vi "test_read-nmea-data2.vi"() -> ()   [LabVIEW 2019] (continued)
F9P\t\t\n15:11:09.78\tF9P\t\t\n15:11:09.80\tF9P\t\t\n15:11:09.82\tF9P\t\t\n15:11:09.84\tF9P\t\t\n15:11:09.86\tF9P\t\t\n15:11:09.88\tF9P\t\t\n15:11:09.90\tF9P\t\t\n15:11:09.92\tF9P\t\t\n15:11:09.94\tF9P\t\t\n15:11:09.96\tF9P\t\t\n15:11:09.98\tF9P\t\t\n15:11:10.00\tF9P\t\t\n15:11:10.02\tF9P\t\t\n15:11:10.04\tF9P\t\t\n15:11:10.06\tF9P\t\t\n15:11:10.08\tF9P\t\t\n15:11:10.10\tF9P\t\t\n15:11:10.12\tF9P\t\t\n15:11:10.14\tF9P\t\t\n15:11:10.16\tF9P\t\t\n15:11:10.18\tF9P\t\t\n15:11:10.20\tF9P\t\t\n15:11:10.22\tF9P\t\t\n15:11:10.24\tF9P\t\t\n15:11:10.26\tF9P\t$GNRMC,061112.00,A,3723.54417,N,12656.89832,E,2.532,132.14,250720,,,A,V*06\n\t\n15:11:10.28\tF9P\t$GNVTG,132.14,T,,M,2.532,N,4.690,K,A*2B\n\t\n15:11:10.30\tF9P\t$GNGGA,061112.00,3723.54417,N,12656.89832,E,1,12,0.68,52.3,M,18.5,M,,*7A\n\t\n15:11:10.32\tF9P\t$GNGSA,A,3,12,06,19,05,17,09,02,,,,,,1.27,0.68,1.08,1*07\n\t\n15:11:10.34\tF9P\t$GNGSA,A,3,85,71,84,,,,,,,,,,1.27,0.68,1.08,2*06\n\t\n15:11:10.36\tF9P\t$GNGSA,A,3,36,19,11,04,09,12,,,,,,,1.27,0.68,1.08,3*03\n\t\n15:11:10.38\tF9P\t$GNGSA,A,3,14,11,33,,,,,,,,,,1.27,0.68,1.08,4*02\n\t\n15:11:10.40\tF9P\t$GPGSV,3,1,09,02,54,318,43,04,18,044,20,05,37,247,30,06,64,047,30,1*69\n\t\n15:11:10.42\tF9P\t$GPGSV,3,2,09,09,45,074,27,12,24,277,15,17,33,153,38,19,53,157,29,1*6D\n\t\n15:11:10.44\tF9P\t$GPGSV,3,3,09,25,12,307,19,1*55\n\t\n15:11:10.46\tF9P\t$GPGSV,3,1,09,02,54,318,,04,18,044,,05,37,247,16,06,64,047,16,6*6B\n\t\n15:11:10.48\tF9P\t$GPGSV,3,2,09,09,45,074,18,12,24,277,,17,33,153,19,19,53,157,,6*6A\n\t\n15:11:10.50\tF9P\t$GPGSV,3,3,09,25,12,307,,6*5A\n\t\n15:11:10.52\tF9P\t$GLGSV,2,1,08,69,12,031,,70,72,041,,71,51,205,21,72,03,209,,1*71\n\t\n15:11:10.54\tF9P\t$GLGSV,2,2,08,77,01,326,,84,20,122,12,85,70,065,24,86,36,330,,1*7E\n\t\n15:11:10.56\tF9P\t$GLGSV,2,1,08,69,12,031,,70,72,041,,71,51,205,18,72,03,209,,3*79\n\t\n15:11:10.58\tF9P\t$GLGSV,2,2,08,77,01,326,,84,20,122,16,85,70,065,19,86,36,330,,3*76\n\t\n15:11:10.60\tF9P\t$GAGSV,2,1,08,02,08,297,08,04,66,118,29,09,32,193,20,11,71,358,25,7*7F\n\t\n15:11:10.62\tF9P\t$GAGSV,2,2,08,12,40,102,20,19,26,045,09,25,09,249,,36,25,308,27,7*74\n\t\n15:11:10.64\tF9P\t$GAGSV,2,1,08,02,08,297,,04,66,118,25,09,32,193,,11,71,358,,2*7B\n\t\n15:11:10.66\tF9P\t$GAGSV,2,2,08,12,40,102,21,19,26,045,,25,09,249,,36,25,308,,2*7C\n\t\n15:11:10.68\tF9P\t$GBGSV,1,1,03,11,50,131,27,14,87,138,28,33,60,219,28,1*4A\n\t\n15:11:10.70\tF9P\t$GBGSV,1,1,03,11,50,131,28,14,87,138,25,33,60,219,,3*40\n\t\n15:11:10.72\tF9P\t$GNGLL,3723.54417,N,12656.89832,E,061112.00,A,A*7A\n\t\n15:11:10.74\tF9P\t\t\n15:11:10.76\tF9P\t\t\n15:11:10.78\tF9P\t\t\n15:11:10.80\tF9P\t\t\n15:11:10.82\tF9P\t\t\n15:11:10.84\tF9P\t\t\n15:11:10.86\tF9P\t\t\n15:11:10.88\tF9P\t\t\n15:11:10.90\tF9P\t\t\n15:11:10.92\tF9P\t\t\n15:11:10.94\tF9P\t\t\n15:11:10.96\tF9P\t\t\n15:11:10.98\tF9P\t\t\n15:11:11.00\tF9P\t\t\n15:11:11.02\tF9P\t\t\n15:11:11.04\tF9P\t\t\n15:11:11.06\tF9P\t\t\n15:11:11.08\tF9P\t\t\n15:11:11.10\tF9P\t\t\n15:11:11.12\tF9P\t\t\n15:11:11.14\tF9P\t\t\n15:11:11.16\tF9P\t\t\n15:11:11.18\tF9P\t\t\n15:11:11.20\tF9P\t\t\n15:11:11.22\tF9P\t\t\n15:11:11.24\tF9P\t\t\n15:11:11.26\tF9P\t$GNRMC,061113.00,A,3723.54360,N,12656.89907,E,2.329,127.33,250720,,,A,V*0A\n\t\n15:11:11.28\tF9P\t$GNVTG,127.33,T,,M,2.329,N,4.313,K,A*28\n\t\n15:11:11.30\tF9P\t$GNGGA,061113.00,3723.54360,N,12656.89907,E,1,12,0.68,51.5,M,18.5,M,,*7E\n\t\n15:11:11.32\tF9P\t$GNGSA,A,3,12,06,19,05,17,09,02,,,,,,1.27,0.68,1.08,1*07\n\t\n15:11:11.34\tF9P\t$GNGSA,A,3,85,71,84,,,,,,,,,,1.27,0.68,1.08,2*06\n\t\n15:11:11.36\tF9P\t$GNGSA,A,3,36,19,11,04,09,12,,,,,,,1.27,0.68,1.08,3*03\n\t\n15:11:11.38\tF9P\t$GNGSA,A,3,14,11,33,,,,,,,,,,1.27,0.68,1.08,4*02\n\t\n15:11:11.40\tF9P\t$GPGSV,3,1,09,02,54,318,33,04,18,044,,05,37,247,29,06,64,047,35,1*61\n\t\n15:11:11.42\tF9P\t$GPGSV,3,2,09,09,45,074,26,12,24,277,26,17,33,153,34,19,53,157,29,1*60\n\t\n15:11:11.44\tF9P\t$GPGSV,3,3,09,25,12,307,20,1*5F\n\t\n15:11:11.46\tF9P\t$GPGSV,3,1,09,02,54,318,,04,18,044,,05,37,247,15,06,64,047,13,6*6D\n\t\n15:11:11.48\tF9P\t$GPGSV,3,2,09,09,45,074,18,12,24,277,,17,33,153,19,19,53,157,,6*6A\n\t\n15:11:11.50\tF9P\t$GPGSV,3,3,09,25,12,307,,6*5A\n\t\n15:11:11.52\tF9P\t$GLGSV,2,1,08,69,12,031,,70,72,041,,71,51,205,22,72,03,209,,1*72\n\t\n15:11:11.54\tF9P\t$GLGSV,2,2,08,77,01,326,,84,20,122,12,85,70,065,24,86,36,330,,1*7E\n\t\n15:11:11.56\tF9P\t$GLGSV,2,1,08,69,12,031,,70,72,041,,71,51,205,17,72,03,209,,3*76\n\t\n15:11:11.58\tF9P\t$GLGSV,2,2,08,77,01,326,,84,20,122,19,85,70,065,18,86,36,330,,3*78\n\t\n15:11:11.60\tF9P\t$GAGSV,2,1,08,02,08,297,08,04,66,118,28,09,32,193,22,11,71,358,26,7*7F\n\t\n15:11:11.62\tF9P\t$GAGSV,2,2,08,12,40,102,21,19,26,045,08,25,09,249,,36,25,308,27,7*74\n\t\n15:11:11.64\tF9P\t$GAGSV,2,1,08,02,08,297,,04,66,118,24,09,32,193,,11,71,358,,2*7A\n\t\n15:11:11.66\tF9P\t$GAGSV,2,2,08,12,40,102,21,19,26,045,,25,09,249,,36,25,308,,2*7C\n\t\n15:11:11.68\tF9P\t$GBGSV,1,1,03,11,50,131,27,14,87,138,25,33,60,219,19,1*45\n\t\n15:11:11.70\tF9P\t$GBGSV,1,1,03,11,50,131,27,14,87,138,23,33,60,219,,3*49\n\t\n15:11:11.72\tF9P\t$GNGLL,3723.54360,N,12656.89907,E,061113.00,A,A*7B\n\t\n15:11:11.74\tF9P\t\t\n15:11:11.76\tF9P\t\t\n15:11:11.78\tF9P\t\t\n15:11:11.80\tF9P\t\t\n15:11:11.82\tF9P\t\t\n15:11:11.84\tF9P\t\t\n15:11:11.86\tF9P\t\t\n15:11:11.88\tF9P\t\t\n15:11:11.90\tF9P\t\t\n15:11:11.92\tF9P\t\t\n15:11:11.94\tF9P\t\t\n15:11:11.96\tF9P\t\t\n15:11:11.98\tF9P\t\t\n15:11:12.00\tF9P\t\t\n15:11:12.02\tF9P\t\t\n15:11:12.04\tF9P\t\t\n15:11:12.06\tF9P\t\t\n15:11:12.08\tF9P\t\t\n15:11:12.10\tF9P\t\t\n15:11:12.12\tF9P\t\t\n15:11:12.14\tF9P\t\t\n15:11:12.16\tF9P\t\t\n15:11:12.18\tF9P\t\t\n15:11:12.20\tF9P\t\t\n15:11:12.22\tF9P\t\t\n15:11:12.24\tF9P\t$GNRMC,061114.00,A,3723.54294,N,12656.89983,E,2.476,124.59,250720,,,A,V*09\n\t\n15:11:12.26\tF9P\t$GNVTG,124.59,T,,M,2.476,N,4.586,K,A*20\n\t\n15:11:12.28\tF9P\t$GNGGA,061114.00,3723.54294,N,12656.89983,E,1,12,0.68,48.6,M,18.5,M,,*74\n\t\n15:11:12.30\tF9P\t$GNGSA,A,3,12,06,19,05,17,09,02,,,,,,1.27,0.68,1.08,1*07\n\t\n15:11:12.32\tF9P\t$GNGSA,A,3,85,71,84,,,,,,,,,,1.27,0.68,1.08,2*06\n\t\n15:11:12.34\tF9P\t$GNGSA,A,3,36,19,11,04,09,12,,,,,,,1.27,0.68,1.08,3*03\n\t\n15:11:12.36\tF9P\t$GNGSA,A,3,14,11,33,,,,,,,,,,1.27,0.68,1.08,4*02\n\t\n15:11:12.38\tF9P\t$GPGSV,3,1,09,02,54,318,40,04,18,044,19,05,37,247,29,06,64,047,37,1*6F\n\t\n15:11:12.40\tF9P\t$GPGSV,3,2,09,09,45,074,27,12,24,277,25,17,33,153,37,19,53,157,31,1*68\n\t\n15:11:12.42\tF9P\t$GPGSV,3,3,09,25,12,307,19,1*55\n\t\n15:11:12.44\tF9P\t$GPGSV,3,1,09,02,54,318,,04,18,044,,05,37,247,14,06,64,047,,6*6E\n\t\n15:11:12.46\tF9P\t$GPGSV,3,2,09,09,45,074,20,12,24,277,,17,33,153,18,19,53,157,,6*60\n\t\n15:11:12.48\tF9P\t$GPGSV,3,3,09,25,12,307,,6*5A\n\t\n15:11:12.50\tF9P\t$GLGSV,2,1,08,69,12,031,,70,72,041,,71,51,205,21,72,03,209,,1*71\n\t\n15:11:12.52\tF9P\t$GLGSV,2,2,08,77,01,326,,84,20,122,13,85,70,065,29,86,36,330,,1*72\n\t\n15:11:12.54\tF9P\t$GLGSV,2,1,08,69,12,031,,70,72,041,,71,51,205,15,72,03,209,,3*74\n\t\n15:11:12.56\tF9P\t$GLGSV,2,2,08,77,01,326,,84,20,122,22,85,70,065,18,86,36,330,,3*70\n\t\n15:11:12.58\tF9P\t$GAGSV,2,1,08,02,08,297,11,04,66,118,27,09,32,193,23,11,71,358,25,7*7A\n\t\n15:11:12.60\tF9P\t$GAGSV,2,2,08,12,40,102,23,19,26,045,14,25,09,249,,36,25,308,33,7*7E\n\t\n15:11:12.62\tF9P\t$GAGSV,2,1,08,02,08,297,,04,66,118,23,09,32,193,,11,71,358,,2*7D\n\t\n15:11:12.64\tF9P\t$GAGSV,2,2,08,12,40,102,21,19,26,045,,25,09,249,,36,25,308,,2*7C\n\t\n15:11:12.66\tF9P\t$GBGSV,1,1,03,11,50,131,25,14,87,138,24,33,60,219,21,1*4D\n\t\n15:11:12.68\tF9P\t$GBGSV,1,1,03,11,50,131,28,14,87,138,21,33,60,219,,3*44\n\t\n15:11:12.70\tF9P\t$GNGLL,3723.54294,N,12656.89983,E,061114.00,A,A*7A\n\t\n15:11:12.72\tF9P\t\t\n15:11:12.74\tF9P\t\t\n15:11:12.76\tF9P\t\t\n15:11:12.78\tF9P\t\t\n15:11:12.80\tF9P\t\t\n15:11:12.82\tF9P\t\t\n15:11:12.84\tF9P\t\t\n15:11:12.86\tF9P\t\t\n15:11:12.88\tF9P\t\t\n15:11:12.90\tF9P\t\t\n15:11:12.92\tF9P\t\t\n15:11:12.94\tF9P\t\t\n15:11:12.96\tF9P\t\t\n15:11:12.98\tF9P\t\t\n15:11:13.00\tF9P\t\t\n15:11:13.02\tF9P\t\t\n15:11:13.04\tF9P\t\t\n15:11:13.06\tF9P\t\t\n15:11:13.08\tF9P\t\t\n15:11:13.10\tF9P\t\t\n15:11:13.12\tF9P\t\t\n15:11:13.14\tF9P\t\t\n15:11:13.16\tF9P\t\t\n15:11:13.18\tF9P\t\t\n15:11:13.20\tF9P\t\t\n15:11:13.22\tF9P\t\t\n15:11:13.24\tF9P\t$GNRMC,061115.00,A,3723.54238,N,12656.90043,E,2.405,126.35,250720,,,A,V*0F\n\t\n15:11:13.26\tF9P\t$GNVTG,126.35,T,,M,2.405,N,4.454,K,A*22\n\t\n15:11:13.28\tF9P\t$GNGGA,061115.00,3723.54238,N,12656.90043,E,1,12,0.68,48.4,M,18.5,M,,*7C\n\t\n15:11:13.30\tF9P\t$GNGSA,A,3,12,06,19,05,17,09,02,,,,,,1.27,0.68,1.08,1*07\n\t\n15:11:13.32\tF9P\t$GNGSA,A,3,85,71,84,,,,,,,,,,1.27,0.68,1.08,2*06\n\t\n15:11:13.34\tF9P\t$GNGSA,A,3,36,19,11,04,09,12,,,,,,,1.27,0.68,1.08,3*03\n\t\n15:11:13.36\tF9P\t$GNGSA,A,3,14,11,33,,,,,,,,,,1.27,0.68,1.08,4*02\n\t\n15:11:13.38\tF9P\t$GPGSV,3,1,09,02,54,318,38,04,18,044,17,05,37,247,31,06,64,047,31,1*61\n\t\n15:11:13.40\tF9P\t$GPGSV,3,2,09,09,45,074,27,12,24,277,23,17,33,153,33,19,53,157,30,1*6B\n\t\n15:11:13.42\tF9P\t$GPGSV,3,3,09,25,12,307,17,1*5B\n\t\n15:11:13.44\tF9P\t$GPGSV,3,1,09,02,54,318,,04,18,044,,05,37,247,,06,64,047,,6*6B\n\t\n15:11:13.46\tF9P\t$GPGSV,3,2,09,09,45,074,19,12,24,277,,17,33,153,20,19,53,157,,6*61\n\t\n15:11:13.48\tF9P\t$GPGSV,3,3,09,25,12,307,,6*5A\n\t\n15:11:13.50\tF9P\t$GLGSV,2,1,08,69,12,031,,70,72,041,,71,51,205,21,72,03,209,,1*71\n\t\n15:11:13.52\tF9P\t$GLGSV,2,2,08,77,01,326,,84,20,122,11,85,70,065,28,86,36,330,,1*71\n\t\n15:11:13.54\tF9P\t$GLGSV,2,1,08,69,12,031,,70,72,041,,71,51,205,13,72,03,209,,3*72\n\t\n15:11:13.56\tF9P\t$GLGSV,2,2,08,77,01,326,,84,20,122,23,85,70,065,20,86,36,330,,3*7A\n\t\n15:11:13.58\tF9P\t$GAGSV,2,1,08,02,08,297,07,04,66,118,27,09,32,193,22,11,71,358,26,7*7F\n\t\n15:11:13.60\tF9P\t$GAGSV,2,2,08,12,40,102,21,19,26,045,13,25,09,249,,36,25,308,32,7*7A\n\t\n15:11:13.62\tF9P\t$GAGSV,2,1,08,02,08,297,,04,66,118,22,09,32,193,,11,71,358,,2*7C\n\t\n15:11:13.64\tF9P\t$GAGSV,2,2,08,12,40,102,19,19,26,045,,25,09,249,,36,25,308,,2*77\n\t\n15:11:13.66\tF9P\t$GBGSV,1,1,03,11,50,131,25,14,87,138,29,33,60,219,27,1*46\n\t\n15:11:13.68\tF9P\t$GBGSV,1,1,03,11,50,131,27,14,87,138,18,33,60,219,,3*41\n\t\n15:11:13.70\tF9P\t$GNGLL,3723.54238,N,12656.90043,E,061115.00,A,A*70\n\t\n15:11:13.72\tF9P\t\t\n15:11:13.74\tF9P\t\t\n15:11:13.76\tF9P\t\t\n15:11:13.78\tF9P\t\t\n15:11:13.80\tF9P\t\t\n15:11:13.82\tF9P\t\t\n15:11:13.84\tF9P\t\t\n15:11:13.86\tF9P\t\t\n15:11:13.88\tF9P\t\t\n15:11:13.90\tF9P\t\t\n15:11:13.92\tF9P\t\t\n15:11:13.94\tF9P\t\t\n15:11:13.96\tF9P\t\t\n15:11:13.98\tF9P\t\t\n15:11:14.00\tF9P\t\t\n15:11:14.02\tF9P\t\t\n15:11:14.04\tF9P\t\t\n15:11:14.06\tF9P\t\t\n15:11:14.08\tF9P\t\t\n15:11:14.10\tF9P\t\t\n15:11:14.12\tF9P\t\t\n15:11:14.15\tF9P\t\t\n15:11:14.17\tF9P\t\t\n15:11:14.19\tF9P\t\t\n15:11:14.21\tF9P\t\t\n15:11:14.23\tF9P\t\t\n15:11:14.25\tF9P\t$GNRMC,061116.00,A,3723.54169,N,12656.90099,E,2.203,129.46,250720,,,A,V*07\n\t\n15:11:14.27\tF9P\t$GNVTG,129.46,T,,M,2.203,N,4.079,K,A*22\n\t\n15:11:14.29\tF9P\t$GNGGA,061116.00,3723.54169,N,12656.90099,E,1,12,0.68,46.9,M,18.5,M,,*7C\n\t\n15:11:14.31\tF9P\t$GNGSA,A,3,12,06,19,05,17,09,02,,,,,,1.27,0.68,1.08,1*07\n\t\n15:11:14.33\tF9P\t$GNGSA,A,3,85,71,84,,,,,,,,,,1.27,0.68,1.08,2*06\n\t\n15:11:14.35\tF9P\t$GNGSA,A,3,36,19,11,04,09,12,,,,,,,1.27,0.68,1.08,3*03\n\t\n15:11:14.37\tF9P\t$GNGSA,A,3,14,11,33,,,,,,,,,,1.27,0.68,1.08,4*02\n\t\n15:11:14.39\tF9P\t$GPGSV,3,1,09,02,54,318,39,04,18,044,17,05,37,247,28,06,64,047,38,1*61\n\t\n15:11:14.41\tF9P\t$GPGSV,3,2,09,09,45,074,27,12,24,277,22,17,33,153,36,19,53,157,25,1*6B\n\t\n15:11:14.43\tF9P\t$GPGSV,3,3,09,25,12,307,18,1*54\n\t\n15:11:14.45\tF9P\t$GPGSV,3,1,09,02,54,318,,04,18,044,,05,37,247,,06,64,047,,6*6B\n\t\n15:11:14.47\tF9P\t$GPGSV,3,2,09,09,45,074,20,12,24,277,,17,33,153,20,19,53,157,,6*6B\n\t\n15:11:14.49\tF9P\t$GPGSV,3,3,09,25,12,307,,6*5A\n\t\n15:11:14.51\tF9P\t$GLGSV,2,1,08,69,12,031,,70,72,041,,71,51,205,20,72,03,209,,1*70\n\t\n15:11:14.53\tF9P\t$GLGSV,2,2,08,77,01,326,,84,20,122,12,85,70,065,31,86,36,330,,1*7A\n\t\n15:11:14.55\tF9P\t$GLGSV,2,1,08,69,12,031,,70,72,041,,71,51,205,15,72,03,209,,3*74\n\t\n15:11:14.57\tF9P\t$GLGSV,2,2,08,77,01,326,,84,20,122,21,85,70,065,21,86,36,330,,3*79\n\t\n15:11:14.59\tF9P\t$GAGSV,2,1,08,02,08,297,09,04,66,118,27,09,32,193,22,11,71,358,25,7*72\n\t\n15:11:14.61\tF9P\t$GAGSV,2,2,08,12,40,102,22,19,26,045,15,25,09,249,,36,25,308,25,7*79\n\t\n15:11:14.63\tF9P\t$GAGSV,2,1,08,02,08,297,,04,66,118,22,09,32,193,,11,71,358,,2*7C\n\t\n15:11:14.65\tF9P\t$GAGSV,2,2,08,12,40,102,21,19,26,045,,25,09,249,,36,25,308,,2*7C\n\t\n15:11:14.67\tF9P\t$GBGSV,1,1,03,11,50,131,24,14,87,138,26,33,60,219,26,1*49\n\t\n15:11:14.69\tF9P\t$GBGSV,1,1,03,11,50,131,27,14,87,138,19,33,60,219,,3*40\n\t\n15:11:14.71\tF9P\t$GNGLL,3723.54169,N,12656.90099,E,061116.00,A,A*73\n\t\n15:11:14.73\tF9P\t\t\n15:11:14.75\tF9P\t\t\n15:11:14.77\tF9P\t\t\n15:11:14.79\tF9P\t\t\n15:11:14.81\tF9P\t\t\n15:11:14.83\tF9P\t\t\n15:11:14.85\tF9P\t\t\n15:11:14.87\tF9P\t\t\n15:11:14.89\tF9P\t\t\n15:11:14.91\tF9P\t\t\n15:11:14.93\tF9P\t\t\n15:11:14.95\tF9P\t\t\n15:11:14.97\tF9P\t\t\n15:11:14.99\tF9P\t\t\n15:11:15.01\tF9P\t\t\n15:11:15.03\tF9P\t\t\n15:11:15.05\tF9P\t\t\n15:11:15.07\tF9P\t\t\n15:11:15.09\tF9P\t\t\n15:11:15.11\tF9P\t\t\n15:11:15.13\tF9P\t\t\n15:11:15.15\tF9P\t\t\n15:11:15.17\tF9P\t\t\n15:11:15.19\tF9P\t\t\n15:11:15.21\tF9P\t\t\n15:11:15.23\tF9P\t\t\n15:11:15.25\tF9P\t$GNRMC,061117.00,A,3723.54104,N,12656.90146,E,2.269,128.78,250720,,,A,V*0E\n\t\n15:11:15.27\tF9P\t$GNVTG,128.78,T,,M,2.269,N,4.202,K,A*2C\n\t\n15:11:15.29\tF9P\t$GNGGA,061117.00,3723.54104,N,12656.90146,E,1,12,0.68,47.4,M,18.5,M,,*79\n\t\n15:11:15.31\tF9P\t$GNGSA,A,3,12,06,19,05,17,09,04,02,,,,,1.27,0.68,1.08,1*03\n\t\n15:11:15.33\tF9P\t$GNGSA,A,3,85,71,84,,,,,,,,,,1.27,0.68,1.08,2*06\n\t\n15:11:15.35\tF9P\t$GNGSA,A,3,36,19,11,04,09,12,,,,,,,1.27,0.68,1.08,3*03\n\t\n15:11:15.37\tF9P\t$GNGSA,A,3,14,11,33,,,,,,,,,,1.27,0.68,1.08,4*02\n\t\n15:11:15.39\tF9P\t$GPGSV,3,1,09,02,54,318,36,04,18,044,17,05,37,247,27,06,64,047,33,1*6A\n\t\n15:11:15.41\tF9P\t$GPGSV,3,2,09,09,45,074,31,12,24,277,22,17,33,153,33,19,53,157,25,1*69\n\t\n15:11:15.43\tF9P\t$GPGSV,3,3,09,25,12,307,19,1*55\n\t\n15:11:15.45\tF9P\t$GPGSV,3,1,09,02,54,318,,04,18,044,,05,37,247,,06,64,047,,6*6B\n\t\n15:11:15.47\tF9P\t$GPGSV,3,2,09,09,45,074,21,12,24,277,,17,33,153,21,19,53,157,,6*6B\n\t\n15:11:15.49\tF9P\t$GPGSV,3,3,09,25,12,307,,6*5A\n\t\n15:11:15.51\tF9P\t$GLGSV,2,1,08,69,12,031,,70,72,041,,71,51,205,20,72,03,209,,1*70\n\t\n15:11:15.53\tF9P\t$GLGSV,2,2,08,77,01,326,,84,20,122,11,85,70,065,25,86,36,330,,1*7C\n\t\n15:11:15.55\tF9P\t$GLGSV,2,1,08,69,12,031,,70,72,041,,71,51,205,15,72,03,209,,3*74\n\t\n15:11:15.57\tF9P\t$GLGSV,2,2,08,77,01,326,,84,20,122,19,85,70,065,19,86,36,330,,3*79\n\t\n15:11:15.59\tF9P\t$GAGSV,2,1,08,02,08,297,10,04,66,118,26,09,32,193,21,11,71,358,25,7*78\n\t\n15:11:15.61\tF9P\t$GAGSV,2,2,08,12,40,102,23,19,26,045,27,25,09,249,,36,25,308,18,7*77\n\t\n15:11:15.63\tF9P\t$GAGSV,2,1,08,02,08,297,,04,66,118,20,09,32,193,,11,71,358,,2*7E\n\t\n15:11:15.65\tF9P\t$GAGSV,2,2,08,12,40,102,,19,26,045,,25,09,249,,36,25,308,,2*7F\n\t\n15:11:15.67\tF9P\t$GBGSV,1,1,03,11,50,131,23,14,87,138,24,33,60,219,25,1*4F\n\t\n15:11:15.69\tF9P\t$GBGSV,1,1,03,11,50,131,26,14,87,138,21,33,60,219,,3*4A\n\t\n15:11:15.71\tF9P\t$GNGLL,3723.54104,N,12656.90146,E,061117.00,A,A*7A\n\t\n15:11:15.73\tF9P\t\t\n15:11:15.75\tF9P\t\t\n15:11:15.77\tF9P\t\t\n15:11:15.79\tF9P\t\t\n15:11:15.81\tF9P\t\t\n15:11:15.83\tF9P\t\t\n15:11:15.85\tF9P\t\t\n15:11:15.87\tF9P\t\t\n15:11:15.89\tF9P\t\t\n15:11:15.91\tF9P\t\t\n15:11:15.93\tF9P\t\t\n15:11:15.95\tF9P\t\t\n15:11:15.97\tF9P\t\t\n15:11:15.99\tF9P\t\t\n15:11:16.01\tF9P\t\t\n15:11:16.03\tF9P\t\t\n15:11:16.05\tF9P\t\t\n15:11:16.07\tF9P\t\t\n15:11:16.09\tF9P\t\t\n15:11:16.11\tF9P\t\t\n15:11:16.13\tF9P\t\t\n15:11:16.15\tF9P\t\t\n15:11:16.17\tF9P\t\t\n15:11:16.19\tF9P\t\t\n15:11:16.21\tF9P\t\t\n15:11:16.23\tF9P\t\t\n15:11:16.25\tF9P\t$GNRMC,061118.00,A,3723.54059,N,12656.90192,E,2.172,128.82,250720,,,A,V*0D\n\t\n15:11:16.27\tF9P\t$GNVTG,128.82,T,,M,2.172,N,4.023,K,A*21\n\t\n15:11:16.29\tF9P\t$GNGGA,061118.00,3723.54059,N,12656.90192,E,1,12,0.68,46.8,M,18.5,M,,*7B\n\t\n15:11:16.31\tF9P\t$GNGSA,A,3,12,06,19,05,17,09,04,02,,,,,1.27,0.68,1.08,1*03\n\t\n15:11:16.33\tF9P\t$GNGSA,A,3,85,71,84,,,,,,,,,,1.27,0.68,1.08,2*06\n\t\n15:11:16.35\tF9P\t$GNGSA,A,3,36,19,11,04,09,12,,,,,,,1.27,0.68,1.08,3*03\n\t\n15:11:16.37\tF9P\t$GNGSA,A,3,14,11,33,,,,,,,,,,1.27,0.68,1.08,4*02\n\t\n15:11:16.39\tF9P\t$GPGSV,3,1,09,02,54,318,30,04,18,044,19,05,37,247,28,06,64,047,31,1*6F\n\t\n15:11:16.41\tF9P\t$GPGSV,3,2,09,09,45,074,30,12,24,277,21,17,33,153,29,19,53,157,23,1*66\n\t\n15:11:16.43\tF9P\t$GPGSV,3,3,09,25,12,307,18,1*54\n\t\n15:11:16.45\tF9P\t$GPGSV,3,1,09,02,54,318,,04,18,044,,05,37,247,,06,64,047,,6*6B\n\t\n15:11:16.47\tF9P\t$GPGSV,3,2,09,09,45,074,22,12,24,277,,17,33,153,22,19,53,157,,6*6B\n\t\n15:11:16.49\tF9P\t$GPGSV,3,3,09,25,12,307,,6*5A\n\t\n15:11:16.51\tF9P\t$GLGSV,2,1,08,69,12,031,,70,72,041,,71,51,205,19,72,03,209,,1*7A\n\t\n15:11:16.53\tF9P\t$GLGSV,2,2,08,77,01,326,,84,20,122,08,85,70,065,25,86,36,330,,1*74\n\t\n15:11:16.55\tF9P\t$GLGSV,2,1,08,69,12,031,,70,72,041,,71,51,205,15,72,03,209,,3*74\n\t\n15:11:16.57\tF9P\t$GLGSV,2,2,08,77,01,326,,84,20,122,18,85,70,065,18,86,36,330,,3*79\n\t\n15:11:16.59\tF9P\t$GAGSV,2,1,08,02,08,297,07,04,66,118,25,09,32,193,21,11,71,358,24,7*7C\n\t\n15:11:16.61\tF9P\t$GAGSV,2,2,08,12,40,102,21,19,26,045,21,25,09,249,,36,25,308,33,7*7A\n\t\n15:11:16.63\tF9P\t$GAGSV,2,1,08,02,08,297,,04,66,118,20,09,32,193,,11,71,358,,2*7E\n\t\n15:11:16.65\tF9P\t$GAGSV,2,2,08,12,40,102,25,19,26,045,,25,09,249,,36,25,308,,2*78\n\t\n15:11:16.67\tF9P\t$GBGSV,1,1,03,11,50,131,24,14,87,138,23,33,60,219,25,1*4F\n\t\n15:11:16.69\tF9P\t$GBGSV,1,1,03,11,50,131,25,14,87,138,22,33,60,219,,3*4A\n\t\n15:11:16.71\tF9P\t$GNGLL,3723.54059,N,12656.90192,E,061118.00,A,A*75\n\t\n15:11:16.73\tF9P\t\t\n15:11:16.75\tF9P\t\t\n15:11:16.77\tF9P\t\t\n15:11:16.79\tF9P\t\t\n15:11:16.81\tF9P\t\t\n15:11:16.83\tF9P\t\t\n15:11:16.85\tF9P\t\t\n15:11:16.87\tF9P\t\t\n15:11:16.89\tF9P\t\t\n15:11:16.91\tF9P\t\t\n15:11:16.93\tF9P\t\t\n15:11:16.95\tF9P\t\t\n15:11:16.97\tF9P\t\t\n15:11:16.99\tF9P\t\t\n15:11:17.01\tF9P\t\t\n15:11:17.03\tF9P\t\t\n15:11:17.05\tF9P\t\t\n15:11:17.07\tF9P\t\t\n15:11:17.09\tF9P\t\t\n15:11:17.11\tF9P\t\t\n15:11:17.13\tF9P\t\t\n15:11:17.15\tF9P\t\t\n15:11:17.17\tF9P\t\t\n15:11:17.19\tF9P\t\t\n15:11:17.21\tF9P\t\t\n15:11:17.23\tF9P\t\t\n15:11:17.25\tF9P\t$GNRMC,061119.00,A,3723.53985,N,12656.90241,E,2.133,136.24,250720,,,A,V*08\n\t\n15:11:17.27\tF9P\t$GNVTG,136.24,T,,M,2.133,N,3.951,K,A*2C\n\t\n15:11:17.29\tF9P\t$GNGGA,061119.00,3723.53985,N,12656.90241,E,1,12,0.68,44.8,M,18.5,M,,*7A\n\t\n15:11:17.31\tF9P\t$GNGSA,A,3,12,06,19,05,17,09,04,02,,,,,1.27,0.68,1.08,1*03\n\t\n15:11:17.33\tF9P\t$GNGSA,A,3,85,71,84,,,,,,,,,,1.27,0.68,1.08,2*06\n\t\n15:11:17.35\tF9P\t$GNGSA,A,3,36,19,11,04,09,12,,,,,,,1.27,0.68,1.08,3*03\n\t\n15:11:17.37\tF9P\t$GNGSA,A,3,14,11,33,,,,,,,,,,1.27,0.68,1.08,4*02\n\t\n15:11:17.39\tF9P\t$GPGSV,3,1,09,02,54,318,27,04,18,044,21,05,37,247,28,06,64,047,32,1*61\n\t\n15:11:17.41\tF9P\t$GPGSV,3,2,09,09,45,074,25,12,24,277,19,17,33,153,36,19,53,157,29,1*6D\n\t\n15:11:17.43\tF9P\t$GPGSV,3,3,09,25,12,307,17,1*5B\n\t\n15:11:17.45\tF9P\t$GPGSV,3,1,09,02,54,318,,04,18,044,,05,37,247,,06,64,047,,6*6B\n\t\n15:11:17.47\tF9P\t$GPGSV,3,2,09,09,45,074,21,12,24,277,,17,33,153,21,19,53,157,,6*6B\n\t\n15:11:17.49\tF9P\t$GPGSV,3,3,09,25,12,307,,6*5A\n\t\n15:11:17.51\tF9P\t$GLGSV,2,1,08,69,12,031,,70,72,041,,71,51,205,19,72,03,209,,1*7A\n\t\n15:11:17.53\tF9P\t$GLGSV,2,2,08,77,01,326,,84,20,122,10,85,70,065,24,86,36,330,,1*7C\n\t\n15:11:17.55\tF9P\t$GLGSV,2,1,08,69,12,031,,70,72,041,,71,51,205,16,72,03,209,,3*77\n\t\n15:11:17.57\tF9P\t$GLGSV,2,2,08,77,01,326,,84,20,122,18,85,70,065,19,86,36,330,,3*78\n\t\n15:11:17.59\tF9P\t$GAGSV,2,1,08,02,08,297,11,04,66,118,24,09,32,193,24,11,71,358,23,7*78\n\t\n15:11:17.61\tF9P\t$GAGSV,2,2,08,12,40,102,22,19,26,045,23,25,09,249,,36,26,308,33,7*78\n\t\n15:11:17.63\tF9P\t
